vi "greater than subvi.vi"(9 "Numeric 3":dbl, 10 "Numeric in":dbl, 11 "Numeric 4":dbl) -> (3 "Numeric out":dbl)   [LabVIEW 2018]
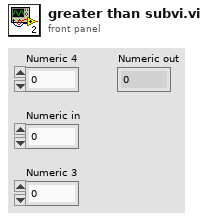
[diagram p1: front panel]
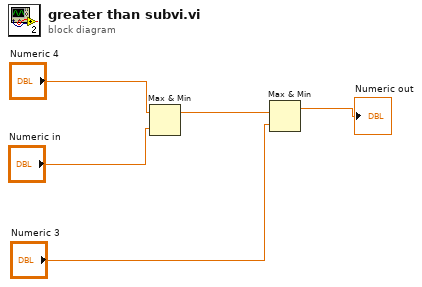
[diagram p0: block diagram]
diagram:
  n1 = Max & Min(x="Numeric 4", y="Numeric in") -> (max(x,y)=w3:dbl)  [unwired: 1 out]
  n2 = Max & Min(x=w3, y="Numeric 3") -> (max(x,y)=→"Numeric out":dbl)  [unwired: 1 out]
